vi "Binary Search on One Hot Encoded Number (U8).vi"(7 "One Hot Encoded Number":u8 format="%08b") -> (8 "Binary Number":u8)   [LabVIEW 2012]
doc: "This VI gives the index the index of first one from LSB. It assumes that the number is one hot encoded.\nInother words it converts one hot encoded number to Binary Number"
panel:
  out "Binary Array":bool[](array[boolean])
  out "a[0]":bool
  out "a[1]":bool
  out "a[2]":bool
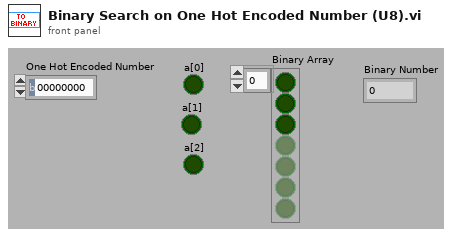
[diagram p1: front panel]
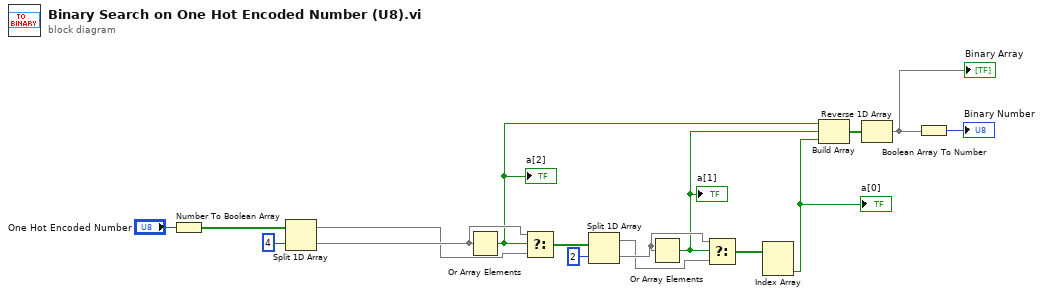
[diagram p0: block diagram]
diagram:
  n1 = Number To Boolean Array(number="One Hot Encoded Number") -> (Boolean array=w1:bool[])
  n2 = Split 1D Array(array=w1, index=4) -> (first subarray=w13:bool[], second subarray=w14:bool[])
  n3 = Or Array Elements(Boolean array=w14) -> (logical OR=w7:bool)
  "a[2]" <- w7
  n4 = Select(t=w14, s=w7, f=w13) -> (s? t:f=w12:bool[])
  n5 = Split 1D Array(array=w12, index=2) -> (first subarray=w9:bool[], second subarray=w10:bool[])
  n6 = Or Array Elements(Boolean array=w10) -> (logical OR=w8:bool)
  "a[1]" <- w8
  n7 = Select(t=w10, s=w8, f=w9) -> (s? t:f=w3:bool[])
  n8 = Index Array(array=w3) -> (element #2=w2:bool)  [unwired: 2 in, 1 out]
  "a[0]" <- w2
  n9 = Build Array(w7, w8, w2) -> (w6:bool[])
  n10 = Reverse 1D Array(array=w6) -> (reversed array=w4:bool[])
  "Binary Array" <- w4
  n11 = Boolean Array To Number(Boolean array=w4) -> (number=→"Binary Number":u8)
